vi "CmdLoadProject.vi"(11 "String":string="project=20200409") -> (3 "loadok":bool)   [LabVIEW 2019]
uses:
  GLB/GLB_Project.vi
  Class/Main Process Class/MPC_VirbVision/Panel RefGlb.vi
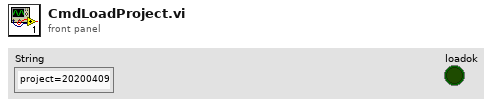
[diagram p1: front panel]
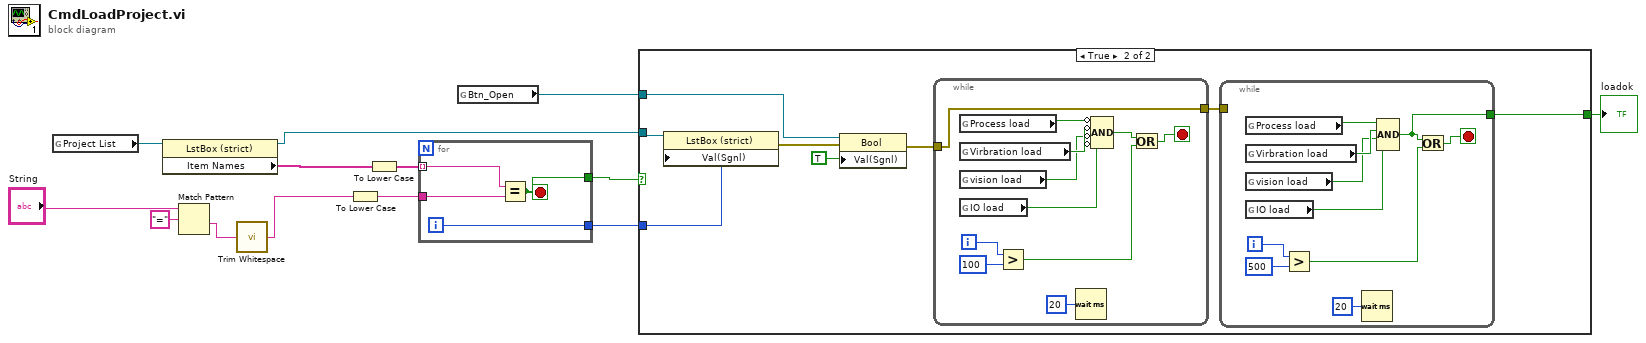
[diagram p0: block diagram]
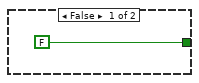
[diagram p2: hidden frame]
diagram:
  n1 = global read "GLB_Project.vi" "Project List"() -> (w10:refnum<vi>)
  n2 = property class="LstBox (strict)"(reference=w10) -> (reference out=w4:refnum<vi>, "Item Names"=w9:string[])  [unwired: 1 in, 1 out]
  n3 = Match Pattern(string="String", regular expression="=") -> (after substring=w11:string)  [unwired: 1 in, 3 out]
  n4 = call <vilib>:"Trim Whitespace.vi"("string"=w11) -> ("trimmed string"=w8:string)  [unwired: 1 in]
  n5 = To Lower Case(string=w8) -> (all lower case string=w7:string)
  n6 = To Lower Case(string=w9) -> (all lower case string=w6:string[])
  n7 = for {
    tunnel: w6 -> [w17] mode=indexing
    tunnel: w7 -> [w16]
    tunnel: [w15] -> w3
    tunnel: [w14] -> w5
    i -> [w15]
    stop <- w14 stop-if-true
    n8 = Equal?(x=w17, y=w16) -> (x = y?=w14:bool)
  }
  n9 = global read "GLB_Project.vi" "Btn_Open"() -> (w2:refnum<vi>)
  n10 = case shown="True" w5 {
    tunnel: w4 -> [_ w26]
    tunnel: w3 -> [_ w25]
    tunnel: w2 -> [_ w24]
    tunnel: [FALSE w21] -> w1
    frame False {
    }
    frame True {
      n11 = property class="LstBox (strict)"(reference=w26, "Val(Sgnl)"=w25) -> (error out=w22:errorcluster)  [unwired: 1 in, 1 out]
      n12 = property class="Bool"(reference=w24, error in=w22, "Val(Sgnl)"=TRUE) -> (error out=w20:errorcluster)  [unwired: 1 out]
      n13 = while {
        tunnel: w20 -> [w27]
        tunnel: [w27] -> w19
        i -> [w33]
        stop <- w30 stop-if-true
        n14 = global read "Panel RefGlb.vi" "Process load"() -> (w37:bool)
        n15 = global read "Panel RefGlb.vi" "Virbration load"() -> (w36:bool)
        n16 = global read "Panel RefGlb.vi" "vision load"() -> (w35:bool)
        n17 = global read "Panel RefGlb.vi" "IO load"() -> (w34:bool)
        n18 = Greater?(x=w33, y=100) -> (0:w28:bool)
        n19 = Wait (ms)(milliseconds to wait=u32 20) -> ()  [unwired: 1 out]
        n20 = Compound Arithmetic op=AND(invert w37, invert w36, invert w35, invert w34) -> (w29:bool)
        n21 = Or(x=w29, y=w28) -> (x .or. y?=w30:bool)
      }
      n22 = while {
        tunnel: [w38] -> w21
        tunnel: w19 -> [_]
        i -> [w43]
        stop <- w39 stop-if-true
        n23 = global read "Panel RefGlb.vi" "Process load"() -> (w47:bool)
        n24 = global read "Panel RefGlb.vi" "Virbration load"() -> (w46:bool)
        n25 = global read "Panel RefGlb.vi" "vision load"() -> (w45:bool)
        n26 = global read "Panel RefGlb.vi" "IO load"() -> (w44:bool)
        n27 = Greater?(x=w43, y=500) -> (0:w40:bool)
        n28 = Wait (ms)(milliseconds to wait=u32 20) -> ()  [unwired: 1 out]
        n29 = Compound Arithmetic op=AND(w47, w46, w45, w44) -> (w38:bool)
        n30 = Or(x=w38, y=w40) -> (x .or. y?=w39:bool)
      }
    }
  }
  "loadok" <- w1
